vi "Conv_GyroDegrees_Heading.vi"(10 "GyroDegrees":dbl) -> (2 "HeadingDegrees":dbl)   [LabVIEW 2019, in "Trajectory_Library.lvlib"]
doc: "Convert angle (radians) to heading (+/- PI ) (radians)\n\nNOTE: gyro increments clockwise. Headings increment counterclockwise. (NOTE: Be careful to check the rotation of your gyro before using this routine to adjust it.)"
uses:
  Trajectory_Library.lvlib
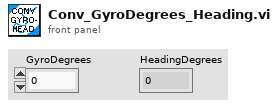
[diagram p1: front panel]
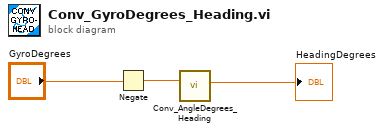
[diagram p0: block diagram]
diagram:
  n1 = Negate(x="GyroDegrees") -> (-x=w2:dbl)
  n2 = call "Conv_AngleDegrees_Heading.vi"("Degrees"=w2) -> ("Heading Degrees"=→"HeadingDegrees":dbl)  [unwired: 10 in]
